vi "Point&Path@Pallet2D__Parameter.vi"(1 "ParamterIn":string) -> (0 "ParamterOut":string)   [LabVIEW 2020]
panel:
  in  "Y Number":string(combo)
  in  "X Number":string(combo)
  in  "PointName":string(combo)
  in  "Confirm":bool
  # "Point&Path@Pallet2D $Point,$X Number,$Y Number\n$Point[0]=Org\n$Point[1]=X End\n$Point[2]=Y End"
  # "X"
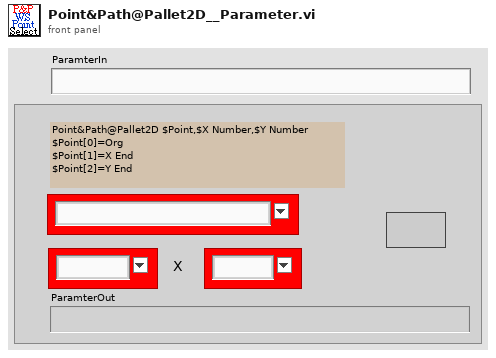
[diagram p1: front panel]
types:
  T1 = enum16{"Get", "UpdatePointS", "Init", "UpdateIndex", "GetCurrent&Index+1", "GetWithIndex", "ChkLast", "GetCurrent"}
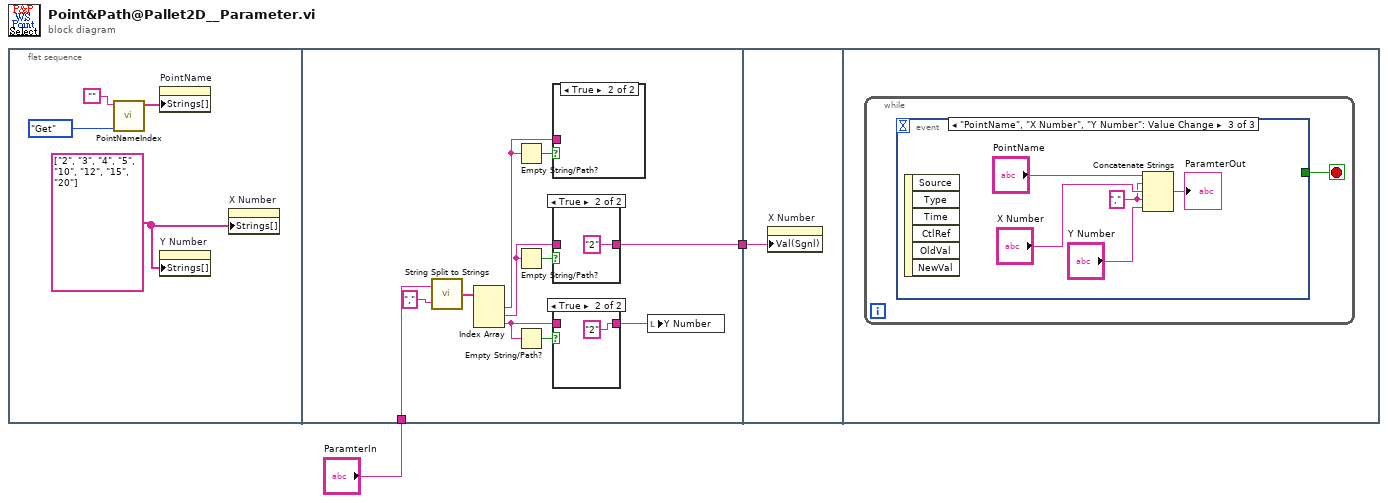
[diagram p0: block diagram]
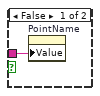
[diagram p4: hidden frame]
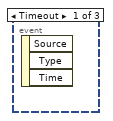
[diagram p5: hidden frame]
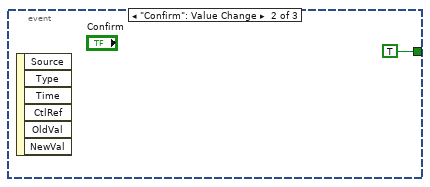
[diagram p6: hidden frame]
diagram:
  n1 = flat-sequence {
    tunnel: "ParamterIn" -> [w14]
    tunnel: [w15] -> w1
    tunnel: w1 -> [w23]
    frame #0 {
      w3 = string[] ["2", "3", "4", "5", "10", "12", "15", "20"] ("Strings []")
      n2 = call "PointNameIndex.vi"("OP"=T1."Get", "PointName"="") -> ("PointNameList"=w4:string[])  [unwired: 4 in, 5 out]
      n3 = property on="PointName" class="CmbBox"("Strings[]"=w4) -> ()  [unwired: 2 in, 2 out]
      n4 = property on="Y Number" class="CmbBox"("Strings[]"=w3) -> ()  [unwired: 2 in, 2 out]
      n5 = property on="X Number" class="CmbBox"("Strings[]"=w3) -> ()  [unwired: 2 in, 2 out]
    }
    frame #1 {
      n6 = call "String Split to Strings.vi"("search string/char (-)"=",", "String"=w14) -> ("Array"=w12:string[])
      n7 = Index Array(array=w12) -> (element #1=w11:string, element #2=w10:string, element #3=w8:string)  [unwired: 3 in]
      n8 = Empty String/Path?(string/path=w11) -> (empty?=w17:bool)
      n9 = Empty String/Path?(string/path=w10) -> (empty?=w16:bool)
      n10 = Empty String/Path?(string/path=w8) -> (empty?=w9:bool)
      n11 = case shown="True" w17 {
        tunnel: w11 -> [w22 _]
        frame False {
          n12 = property on="PointName" class="CmbBox"("Value"=w22) -> ()  [unwired: 2 in, 2 out]
        }
        frame True {
        }
      }
      n13 = case shown="True" w16 {
        tunnel: [w20 "2" ("ParamterIn")] -> w15
        tunnel: w10 -> [w20 _]
        frame False {
        }
        frame True {
        }
      }
      n14 = case shown="True" w9 {
        tunnel: [w18 "2" ("ParamterIn")] -> w7
        tunnel: w8 -> [w18 _]
        frame False {
        }
        frame True {
        }
      }
      n15 = local write "Y Number"(w7) -> ()
    }
    frame #2 {
      n16 = property on="X Number" class="CmbBox"("Val(Sgnl)"=w23) -> ()  [unwired: 2 in, 2 out]
    }
    frame #3 {
      n17 = while {
        stop <- w24 stop-if-true
        n18 = event shown="[2] \"PointName\", \"X Number\", \"Y Number\": Value Change" {
          selector: _ -> [_ _ _]
          dyn-events: _ -> [_ _ _]
          timeout: _ -> [_ _ _]
          tunnel: [_ TRUE _] -> w24
          event Timeout {
            n19 = event-data() -> ()  [unwired: 1 in, 3 out]
          }
          event "Confirm": Value Change {
            n20 = event-data() -> ()  [unwired: 1 in, 6 out]
          }
          event "PointName", "X Number", "Y Number": Value Change {
            w27 = ","
            n21 = event-data() -> ()  [unwired: 1 in, 6 out]
            n22 = Concatenate Strings("PointName", w27, "X Number", w27, "Y Number") -> (→"ParamterOut":string)
          }
        }
      }
    }
  }
